vi "MGI SZL List Zip Contents.vi"(8 "Error In":errorcluster, 10 "File Info? (F)":bool, 11 "Zip File":refnum<k24>) -> (0 "Error Out":errorcluster, 1 "File Info[]":T1[](array[typedef]) {"CompressionMethod" items=["Stored"=0, "Deflated"=8, "Deflate64"=9, "BZip2"=11, "WinZipAES"=99]}, 2 "File Name[]":string[](array[string]), 3 "Zip File Out":refnum<k24>)   [LabVIEW 2016]
doc: "Lists the file names of all the files in the zip file and if file info? is true, outputs a large cluster of info about each file.\n\nThis VI relies on the Sharp Zip Library which is a .NET assembly written in C# by Mike Krueger. It is licenced under the GPL with a special exception permitting independent modules to link to the library regardless of the license terms of the independent module. \n\nMore information about the library and its license is available from:\nhttp://www.icsharpcode.net/opensource/sharpziplib/\n\nAuthored by Matthew G. Harrison\nsupport@mooregoodideas.com\nwww.mooregoodideas.com\n\nCopyright (c) 2010, Moore Good Ideas, Inc.\n\nAll rights reserved.\n\nRedistribution and use in source and binary forms, with or without modification, are permitted provided that the following conditions are met:\n\n * Redistributions of source code must retain the above copyright notice, this list of conditions and the following disclaimer.\n * Redistributions in binary form must reproduce the above copyright notice, this list of conditions and the following disclaimer in the documentation and/or other materials provided with the distribution.\n * Neither the name of Moore Good Ideas, Inc. nor the names of its contributors may be used to endorse or promote products derived from this software without specific prior written permission.\n\nTHIS SOFTWARE IS PROVIDED BY THE COPYRIGHT HOLDERS AND CONTRIBUTORS \"AS IS\" AND ANY EXPRESS OR IMPLIED WARRANTIES, INCLUDING, BUT NOT LIMITED TO, THE IMPLIED WARRANTIES OF MERCHANTABILITY AND FITNESS FOR A PARTICULAR PURPOSE ARE DISCLAIMED. IN NO EVENT SHALL THE COPYRIGHT OWNER OR CONTRIBUTORS BE LIABLE FOR ANY DIRECT, INDIRECT, INCIDENTAL, SPECIAL, EXEMPLARY, OR CONSEQUENTIAL DAMAGES (INCLUDING, BUT NOT LIMITED TO, PROCUREMENT OF SUBSTITUTE GOODS OR SERVICES; LOSS OF USE, DATA, OR PROFITS; OR BUSINESS INTERRUPTION) HOWEVER CAUSED AND ON ANY THEORY OF LIABILITY, WHETHER IN CONTRACT, STRICT LIABILITY, OR TORT (INCLUDING NEGLIGENCE OR OTHERWISE) ARISING IN ANY WAY OUT OF THE USE OF THIS SOFTWARE, EVEN IF ADVISED OF THE POSSIBILITY OF SUCH DAMAGE."
uses:
  C:/Program Files (x86)/National Instruments/LabVIEW 2016/user.lib/_MGI/File/Zip/Support Files/ICSharpCode.SharpZipLib.dll
  Support Files/ICSharpCode.SharpZipLib.dll
  <userlib>/_MGI/File/Zip/MGI SZL File Info.ctl
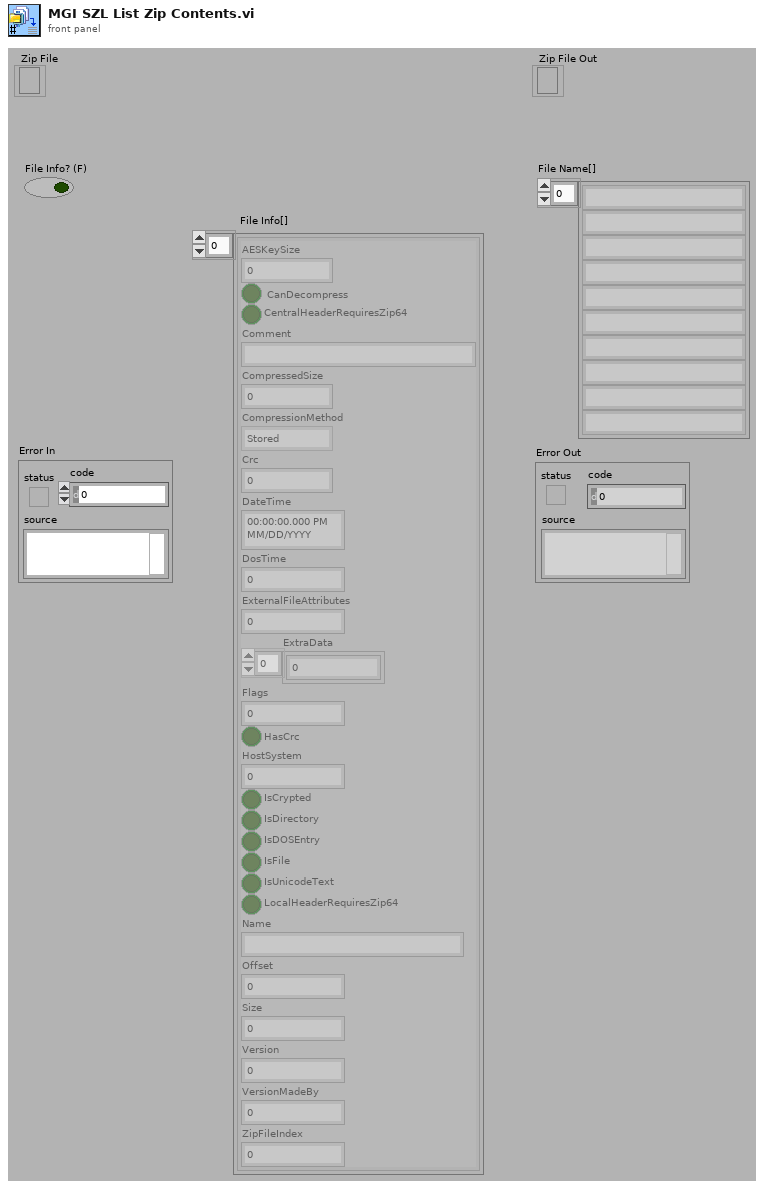
[diagram p1: front panel]
types:
  T1 = typedef "MGI SZL File Info.ctl" = cluster{"AESKeySize":i32, "CanDecompress":bool, "CentralHeaderRequiresZip64":bool, "Comment":string, "CompressedSize":i64, "CompressionMethod":i32, "Crc":i64, "DateTime":timestamp, "DosTime":i64, "ExternalFileAttributes":i32, "ExtraData":u8[], "Flags":i32, "HasCrc":bool, "HostSystem":i32, "IsCrypted":bool, "IsDirectory":bool, "IsDOSEntry":bool, "IsFile":bool, "IsUnicodeText":bool, "LocalHeaderRequiresZip64":bool, "Name":string, "Offset":i64, "Size":i64, "Version":i32, "VersionMadeBy":i32, "ZipFileIndex":i64}
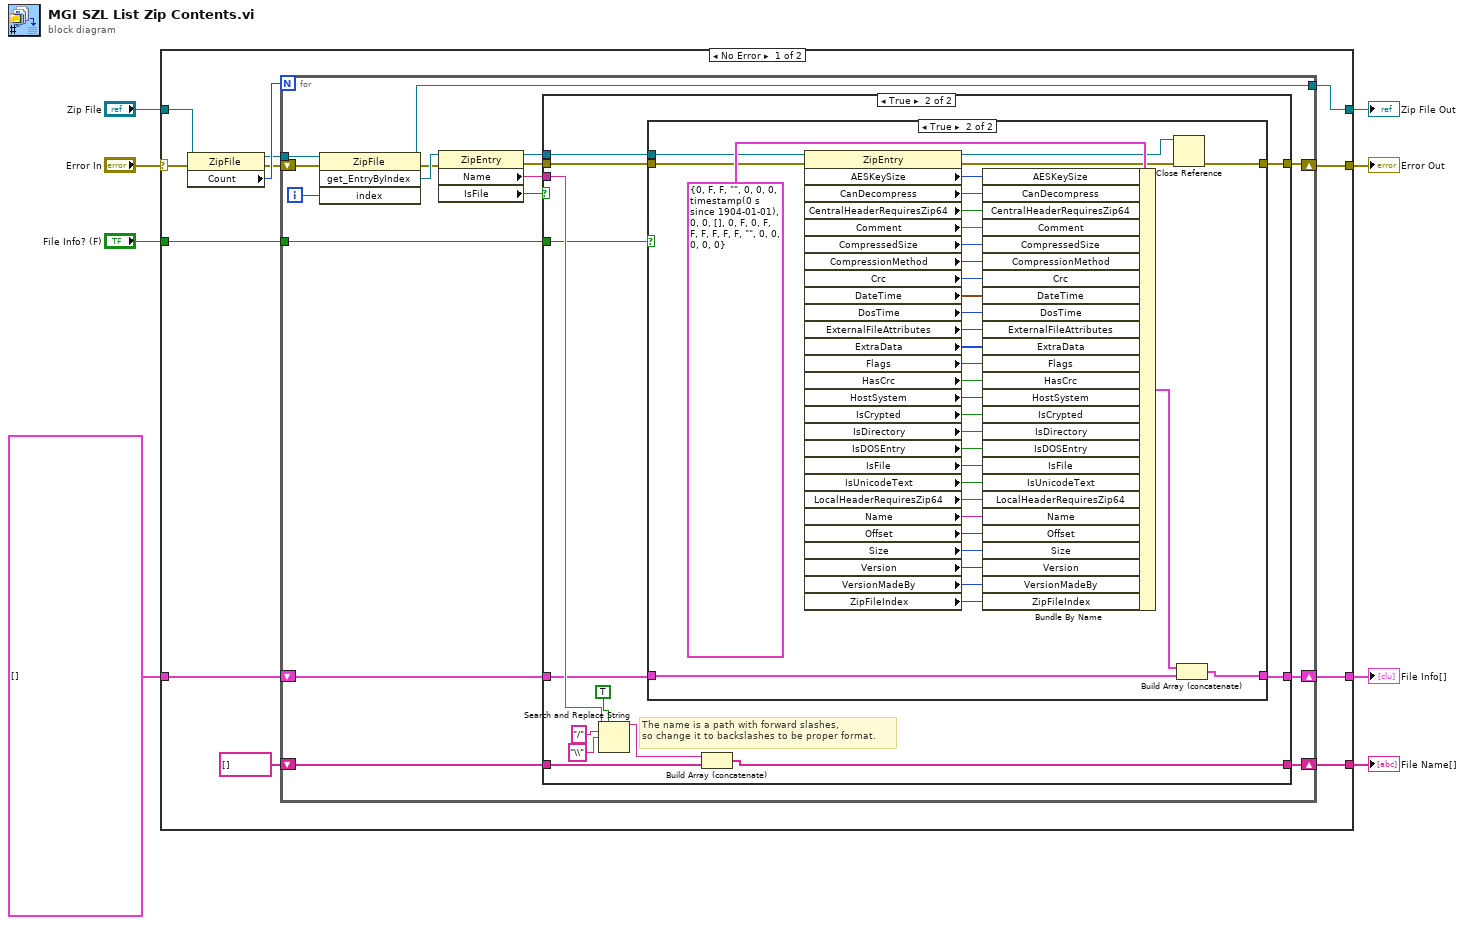
[diagram p0: block diagram]
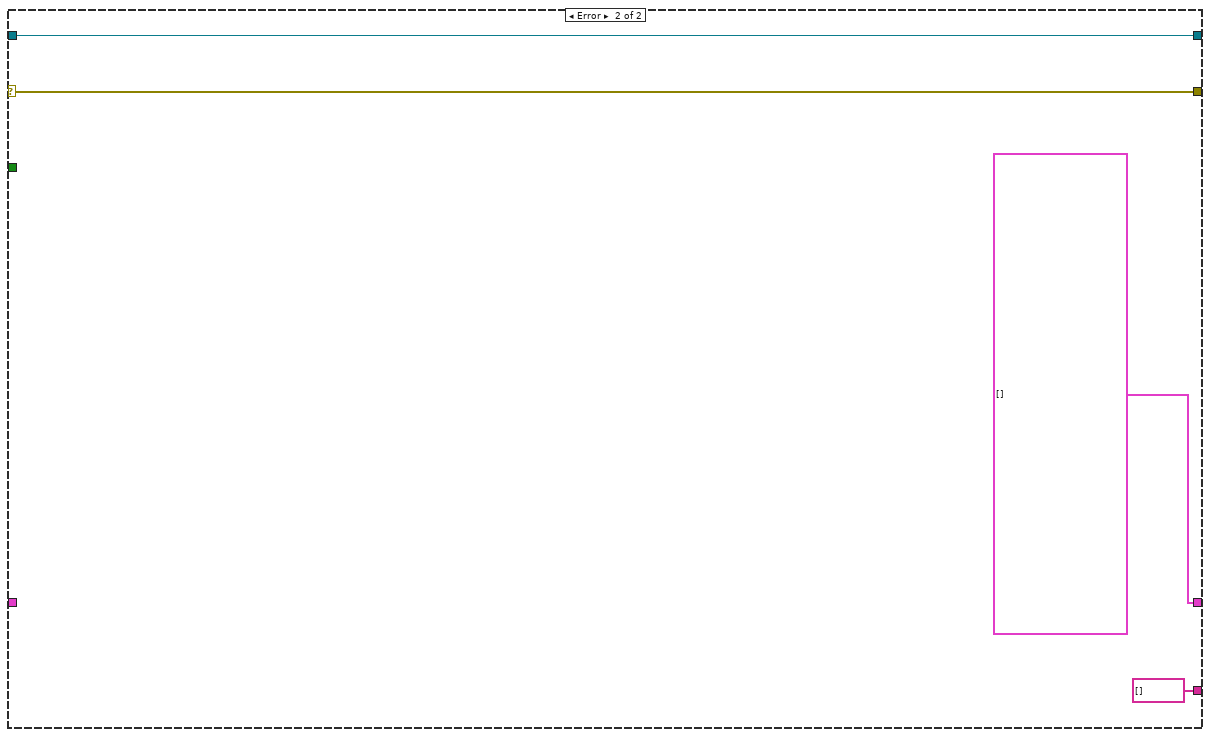
[diagram p4: hidden frame]
diagram:
  n1 = case shown="No Error" "Error In" {
    selector: "Error In" -> [w10 w93]
    tunnel: "Zip File" -> [w20 w92]
    tunnel: "File Info? (F)" -> [w16 _]
    tunnel: [w14 w93] -> w6
    tunnel: [w13 T1[] []] -> w5
    tunnel: [w12 string[] []] -> w4
    tunnel: [w11 w92] -> w3
    tunnel: T1[] [] -> [w9 _]
    frame No Error {
      n2 = property class="ZipFile"(reference=w20, error in=w10) -> (reference out=w18:refnum<k24>, error out=w17:errorcluster, "Count"=w19:i64)
      n3 = for {
        N: w19 -> [_]
        tunnel: w18 -> [w35]
        shift-right: [w28] -> w14
        shift-left: w17 -> [w33]
        tunnel: w16 -> [w30]
        shift-right: [w26] -> w12
        shift-left: string[] [] -> [w25]
        shift-right: [w24] -> w13
        shift-left: w9 -> [w23]
        tunnel: [w22] -> w11
        i -> [w36]
        n4 = invoke class="ZipFile" method="get_EntryByIndex"(reference=w35, error in=w33, "index"=w36) -> (reference out=w22:refnum<k24>, error out=w32:errorcluster, "get_EntryByIndex"=w34:refnum<k24>)  [unwired: 1 in, 1 out]
        n5 = property class="ZipEntry"(reference=w34, error in=w32) -> (reference out=w27:refnum<k24>, error out=w29:errorcluster, "Name"=w31:string, "IsFile"=w21:bool)
        n6 = case shown="True" w21 {
          tunnel: w31 -> [_ w52]
          tunnel: w30 -> [_ w48]
          tunnel: w29 -> [w39 w47]
          tunnel: [w39 w46] -> w28
          tunnel: w27 -> [_ w45]
          tunnel: [w37 w43] -> w26
          tunnel: w25 -> [w37 w42]
          tunnel: [w38 w41] -> w24
          tunnel: w23 -> [w38 w40]
          frame False {
          }
          frame True {
            # "The name is a path with forward slashes,\nso change it to backslashes to be proper format."
            n7 = Search and Replace String(replace all?=TRUE ("replace all? (F)"), input string=w52, search string="/", replace string="\\" ("replace string (\"\")")) -> (result string=w44:string)  [unwired: 4 in, 3 out]
            n8 = case shown="True" w48 {
              tunnel: w47 -> [w54 w62]
              tunnel: [w54 w56] -> w46
              tunnel: w45 -> [_ w61]
              tunnel: [w53 w59] -> w41
              tunnel: w40 -> [w53 w58]
              frame False {
              }
              frame True {
                n9 = property class="ZipEntry"(reference=w61, error in=w62) -> (reference out=w55:refnum<k24>, error out=w57:errorcluster, "AESKeySize"=w88:i32, "CanDecompress"=w87:bool, "CentralHeaderRequiresZip64"=w86:bool, "Comment"=w85:string, "CompressedSize"=w84:i64, "CompressionMethod"=w83:i32, "Crc"=w82:i64, "DateTime"=w81:timestamp, "DosTime"=w80:i64, "ExternalFileAttributes"=w79:i32, "ExtraData"=w78:u8[], "Flags"=w77:i32, "HasCrc"=w76:bool, "HostSystem"=w75:i32, "IsCrypted"=w74:bool, "IsDirectory"=w73:bool, "IsDOSEntry"=w72:bool, "IsFile"=w71:bool, "IsUnicodeText"=w70:bool, "LocalHeaderRequiresZip64"=w69:bool, "Name"=w68:string, "Offset"=w67:i64, "Size"=w66:i64, "Version"=w65:i32, "VersionMadeBy"=w64:i32, "ZipFileIndex"=w63:i64)
                n10 = Bundle By Name(cluster=T1 {"AESKeySize"=0, "CanDecompress"=FALSE, "CentralHeaderRequiresZip64"=FALSE, "Comment"="", "CompressedSize"=0, "CompressionMethod"=0, "Crc"=0, "DateTime"=timestamp(0 s since 1904-01-01), "DosTime"=0, "ExternalFileAttributes"=0, "ExtraData"=[], "Flags"=0, "HasCrc"=FALSE, "HostSystem"=0, "IsCrypted"=FALSE, "IsDirectory"=FALSE, "IsDOSEntry"=FALSE, "IsFile"=FALSE, "IsUnicodeText"=FALSE, "LocalHeaderRequiresZip64"=FALSE, "Name"="", "Offset"=0, "Size"=0, "Version"=0, "VersionMadeBy"=0, "ZipFileIndex"=0} ("file info"), "AESKeySize"=w88, "CanDecompress"=w87, "CentralHeaderRequiresZip64"=w86, "Comment"=w85, "CompressedSize"=w84, "CompressionMethod"=w83, "Crc"=w82, "DateTime"=w81, "DosTime"=w80, "ExternalFileAttributes"=w79, "ExtraData"=w78, "Flags"=w77, "HasCrc"=w76, "HostSystem"=w75, "IsCrypted"=w74, "IsDirectory"=w73, "IsDOSEntry"=w72, "IsFile"=w71, "IsUnicodeText"=w70, "LocalHeaderRequiresZip64"=w69, "Name"=w68, "Offset"=w67, "Size"=w66, "Version"=w65, "VersionMadeBy"=w64, "ZipFileIndex"=w63) -> (w60:T1)
                n11 = Close Reference(reference=w55, error in (no error)=w57) -> (error out=w56:errorcluster)
                n12 = Build Array (concatenate)(w60, w58) -> (w59:T1[])
              }
            }
            n13 = Build Array (concatenate)(w44, w42) -> (w43:string[])
          }
        }
      }
    }
    frame Error {
    }
  }
  "Error Out" <- w6
  "File Info[]" <- w5
  "File Name[]" <- w4
  "Zip File Out" <- w3
